vi "Populate Device Info.vi"(8 "error in":errorcluster, 11 "UI Actor in":refnum<class "UI Actor.lvclass">) -> (0 "error out":errorcluster, 3 "UI Actor out":refnum<class "UI Actor.lvclass">)   [LabVIEW 2024, in "UI Actor.lvlib" / "UI Actor.lvclass"]
uses:
  UI Actor.lvclass
  Controls/Device Info.ctl
  UI Actor.lvclass/UI Actor.ctl
  Core/Device Info/Device Info.lvclass
  Core/EDS/EDS.lvclass
  <vilib>/Utility/Data Type/NI_Data Type.lvlib
  <userlib>/_OpenG.lib/lvdata/lvdata.llb/openg_variant.lvlib
  <vilib>/JDP Science/JDP Science Common Utilities/JDP Utility.lvlib
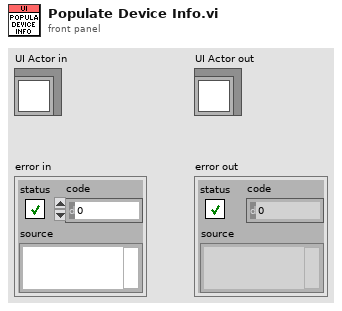
[diagram p1: front panel]
types:
  T1 = typedef "Device Info.ctl" = cluster{"ProductName":string, "ProductNumber":string, "VendorName":string, "VendorNumber":string}
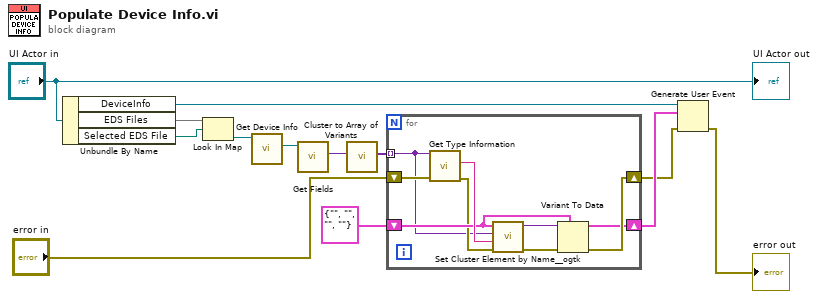
[diagram p0: block diagram]
diagram:
  n1 = Unbundle By Name("UI Actor in") -> ("DeviceInfo"=w12:refnum<user-event>, "EDS Files"=w10:map{path, refnum<class "EDS.lvclass">}, "Selected EDS File"=w8:path)
  n2 = Look In Map(map=w10, key=w8) -> (value=w9:refnum<class "EDS.lvclass">)  [unwired: 1 in, 1 out]
  n3 = call "Get Device Info.vi"("EDS in"=w9) -> ("Device Info"=w7:refnum<class "Device Info.lvclass">)  [unwired: 9 in, 1 out]
  n4 = call-dynamic "Get Fields.vi"("Device Info in"=w7) -> ("Fields Cluster"=w1:variant)  [unwired: 9 in, 1 out]
  n5 = call <vilib>:"Cluster to Array of Variants.vi"("Cluster"=w1) -> ("Array of Cluster Elements"=w3:variant[])  [unwired: 10 in]
  n6 = for {
    tunnel: w3 -> [w14] mode=indexing
    shift-right: [w17] -> w5
    shift-left: T1 {"ProductName"="", "ProductNumber"="", "VendorName"="", "VendorNumber"=""} ("DeviceInfo") -> [w18]
    shift-right: [w20] -> w4
    shift-left: "error in" -> [w16]
    n7 = call <vilib>:"Get Type Information.vi"("error in (no error)"=w16, "variant"=w14) -> ("error out"=w15:errorcluster, "name"=w22:string)  [unwired: 5 in, 3 out]
    n8 = call <userlib>:"Set Cluster Element by Name__ogtk.vi"("error in (no error)"=w15, "Element Name (\"\": New Element Data Name)"=w22, "New Element Value"=w14, "Cluster"=w18) -> ("error out"=w21:errorcluster, "VCluster out"=w19:variant)  [unwired: 5 in, 1 out]
    n9 = Variant To Data(error in=w21, type=w18, Variant=w19) -> (data=w17:T1, error out=w20:errorcluster)
  }
  n10 = Generate User Event(user event=w12, event data cluster=w5, error in=w4) -> (error out=→"error out":errorcluster)  [unwired: 1 in, 1 out]
  "UI Actor out" <- "UI Actor in"
